vi "WaitForEventBack.vi"(8 "error in (no error)":errorcluster, 9 "TimeOut":i32=-1, 11 "CONTROLLER in":refnum<class "CONTROLLER.lvclass">) -> (0 "error out":errorcluster, 3 "CONTROLLER out":refnum<class "CONTROLLER.lvclass">)   [LabVIEW 2013, in "CONTROLLER.lvclass"]
uses:
  CONTROLLER.lvclass
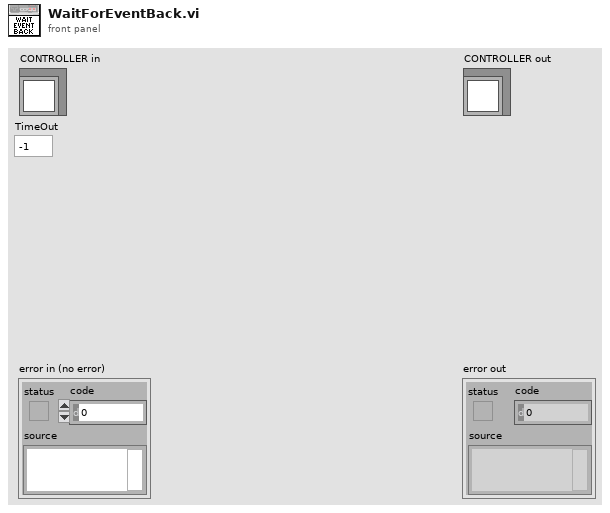
[diagram p1: front panel]
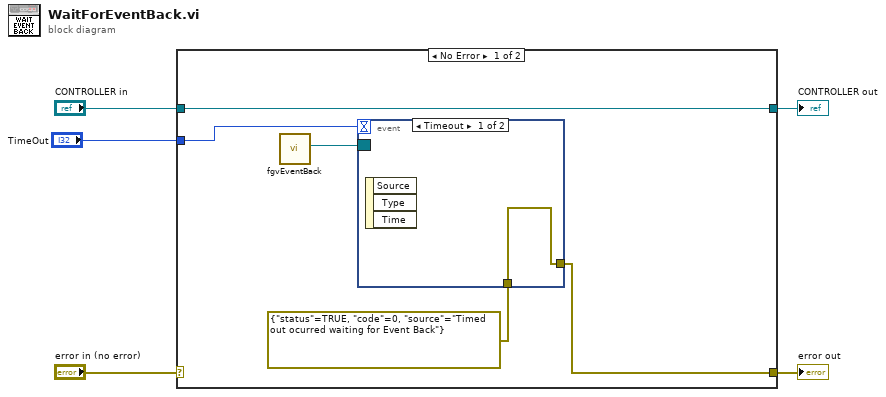
[diagram p0: block diagram]
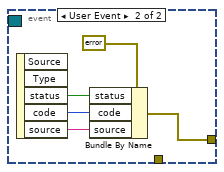
[diagram p2: hidden frame]
diagram:
  n1 = case shown="No Error" "error in (no error)" {
    selector: "error in (no error)" -> [_ w18]
    tunnel: [w8 w18] -> w4
    tunnel: [w10 w17] -> w2
    tunnel: "CONTROLLER in" -> [w10 w17]
    tunnel: "TimeOut" -> [w7 _]
    frame No Error {
      n2 = call "fgvEventBack.vi"() -> ("EventRefNum out"=w9:refnum<event-registration>)  [unwired: 9 in, 2 out]
      n3 = event shown="[0] Timeout" {
        selector: w9 -> [_ _]
        dyn-events: _ -> [_ _]
        timeout: w7 -> [_ _]
        tunnel: [w11 w12] -> w8
        tunnel: errorcluster {"status"=TRUE, "code"=0, "source"="Timed out ocurred waiting for Event Back"} ("error out") -> [w11 _]
        event Timeout {
          n4 = event-data() -> ()  [unwired: 1 in, 3 out]
        }
        event User Event {
          n5 = event-data() -> ("status"=w15:bool, "code"=w14:i32, "source"=w13:string)  [unwired: 1 in, 2 out]
          n6 = Bundle By Name(cluster=errorcluster {"status"=FALSE, "code"=0, "source"=""} ("error out"), "status"=w15, "code"=w14, "source"=w13) -> (w12:errorcluster)
        }
      }
    }
    frame Error {
    }
  }
  "error out" <- w4
  "CONTROLLER out" <- w2
